vi "Check For Internet Connection to WIKI.vi"() -> (0 "error out":errorcluster, 2 "Connected to internet?":bool)   [LabVIEW 2015]
panel:
  out "standard output":string
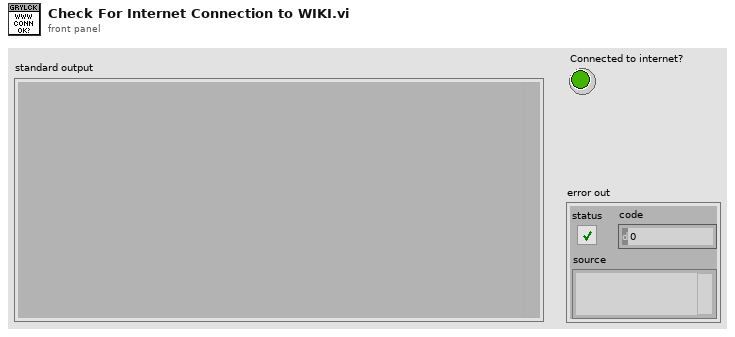
[diagram p1: front panel]
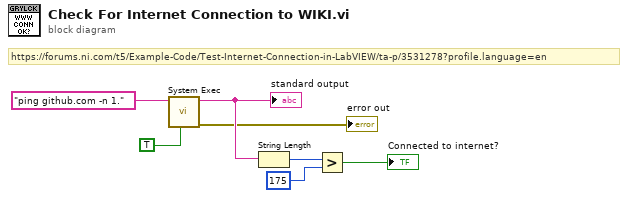
[diagram p0: block diagram]
diagram:
  # "https://forums.ni.com/t5/Example-Code/Test-Internet-Connection-in-LabVIEW/ta-p/3531278?profile.language=en"
  n1 = call <vilib>:"System Exec.vi"("run minimized? (F)"=TRUE, "command line"="ping github.com -n 1.") -> ("error out"=→"error out":errorcluster, "standard output"=w7:string)  [unwired: 6 in, 2 out]
  "standard output" <- w7
  n2 = String Length(string=w7) -> (length=w6:i32)
  n3 = Greater?(x=w6, y=175) -> (0:→"Connected to internet?":bool)
